vi "DWF MSO Query Digital Channel.vi"(0 "Instrument Handle In":u32, 7 "Channel":string, 11 "Error In":errorcluster caption="Error In (no error)") -> (4 "Instrument Handle Out":u32, 6 "Channel Enabled":bool, 15 "Error Out":errorcluster)   [LabVIEW 2015, in "DigilentWF.lvlib"]
doc: "Indicates whether the specified digital channel is enabled."
uses:
  <vilib>/DigilentWF/DigilentWF.lvlib
  dwf.dll
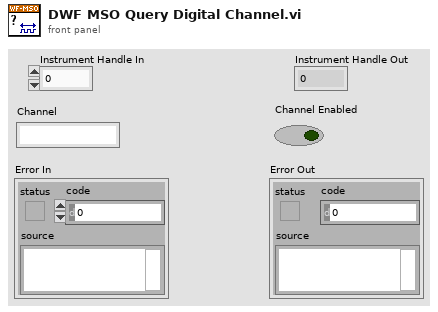
[diagram p1: front panel]
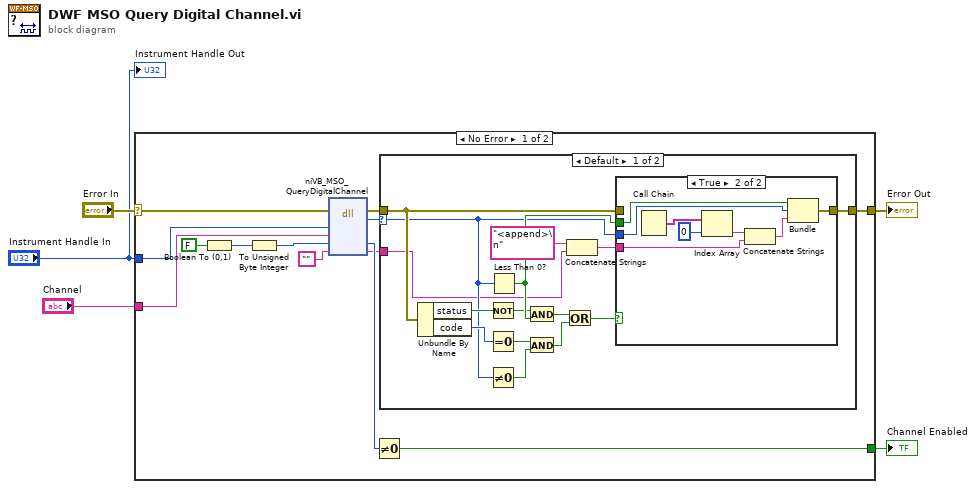
[diagram p0: block diagram]
diagram:
  n1 = case "outter_case" shown="No Error" "Error In" {
    selector: "Error In" -> [w18 w44]
    tunnel: [w15 w44] -> w4
    tunnel: "Instrument Handle In" -> [w14 _]
    tunnel: "Channel" -> [w13 _]
    tunnel: [w9 _] -> w2
    frame No Error {
      n2 = Boolean To (0,1)(Boolean=FALSE ("Channel Enabled")) -> (0, 1=w12:i16)
      n3 = To Unsigned Byte Integer(number=w12) -> (unsigned 8bit integer=w10:u8)
      n4 = dll-call lib="dwf.*" fn="niVB_MSO_QueryDigitalChannel"(error in=w18, "InstrumentHandle"=w14, "Channel"=w13, "ChannelEnabled"=w10, "szError"="") -> (error out=w17:errorcluster, "return type"=w16:i32, "ChannelEnabled"=w8:u8, "szError"=w6:string)  [unwired: 4 in, 1 out]
      n5 = Not Equal To 0?(x=w8) -> (x != 0?=w9:bool)
      n6 = case "inner_case" shown="Default" w16 {
        selector: w16 -> [w23 _]
        tunnel: w17 -> [w24 w43]
        tunnel: [w20 w43] -> w15
        tunnel: w6 -> [w19 _]
        frame Default {
          n7 = Unbundle By Name(w24) -> ("status"=w28:bool, "code"=w32:i32)
          n8 = Not(x=w28) -> (.not. x?=w31:bool)
          n9 = Equal To 0?(x=w32) -> (x = 0?=w27:bool)
          n10 = Not Equal To 0?(x=w23) -> (x != 0?=w30:bool)
          n11 = Less Than 0?(x=w23) -> (x < 0?=w33:bool)
          n12 = And(x=w31, y=w33) -> (x .and. y?=w29:bool)
          n13 = And(x=w27, y=w30) -> (x .and. y?=w26:bool)
          n14 = Or(x=w29, y=w26) -> (x .or. y?=w25:bool)
          n15 = Concatenate Strings("<append>\n" ("string"), w19) -> (w22:string)
          n16 = case shown="True" w25 {
            tunnel: [w34 w41] -> w20
            tunnel: w23 -> [_ w40]
            tunnel: w33 -> [_ w39]
            tunnel: w24 -> [w34 _]
            tunnel: w22 -> [_ w35]
            frame False {
            }
            frame True {
              n17 = Call Chain() -> (call chain=w38:string[])
              n18 = Index Array(array=w38, index=0) -> (element=w37:string)
              n19 = Concatenate Strings(w37, w35) -> (w42:string)
              n20 = Bundle(w39, "return type"=w40, w42) -> (w41:cluster{bool, "return type":i32, string})  [unwired: 1 out]
            }
          }
        }
        frame 0 {
        }
      }
    }
    frame Error {
    }
  }
  "Error Out" <- w4
  "Channel Enabled" <- w2
  "Instrument Handle Out" <- "Instrument Handle In"
